vi "publishStatus.vi"(8 "error in (no error)":errorcluster, 10 "DeviceStatus":T1, 11 "MonoCommunicator in":refnum<class "MonoCommunicator.lvclass">) -> (0 "error out":errorcluster, 3 "MonoCommunicator out":refnum<class "MonoCommunicator.lvclass">)   [LabVIEW 2016, in "MonoCommunicator.lvclass"]
uses:
  MonoCommunicator.lvclass
  Typedefs/DeviceStatus.ctl
  Typedefs/publishers.ctl
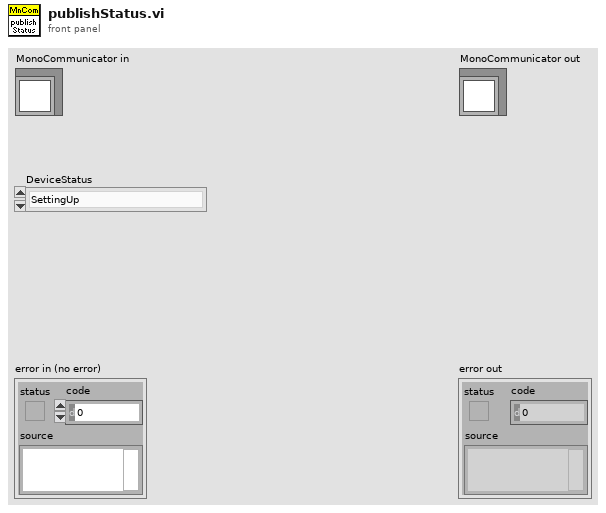
[diagram p1: front panel]
types:
  T1 = typedef "DeviceStatus.ctl" = enum16{"SettingUp", "Ready", "Offline", "Fault"}
  T2 = typedef "publishers.ctl" = enum16{"Wavelength", "Grating", "FrontEntranceSlitPosition", "FrontExitSlitPosition", "SoftwareStatus", "MonochromatorId", "Ack"}
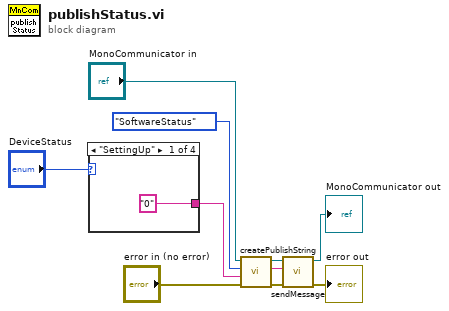
[diagram p0: block diagram]
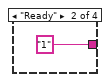
[diagram p2: hidden frame]
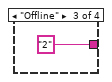
[diagram p3: hidden frame]
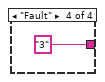
[diagram p4: hidden frame]
diagram:
  n1 = case shown="\"SettingUp\"" "DeviceStatus" {
    tunnel: ["0" "1" "2" "3"] -> w1
    frame "SettingUp" {
    }
    frame "Ready" {
    }
    frame "Offline" {
    }
    frame "Fault" {
    }
  }
  n2 = call "createPublishString.vi"("error in (no error)"="error in (no error)", "parameter"=w1, "publishers"=publishers."SoftwareStatus", "MonoCommunicator in"="MonoCommunicator in") -> ("error out"=w7:errorcluster, "string"=w8:string, "MonoCommunicator out"=w9:refnum<class "MonoCommunicator.lvclass">)  [unwired: 5 in]
  n3 = call-dynamic "sendMessage.vi"("error in (no error)"=w7, "message"=w8, "MonoCommunicator in"=w9) -> ("error out"=→"error out":errorcluster, "MonoCommunicator out"=→"MonoCommunicator out":refnum<class "MonoCommunicator.lvclass">)  [unwired: 7 in]
